vi "Queue_Enqueue.vi"(6 "data":variant, 7 "timeout (-1)":i32=-1, 9 "cmd":string, 10 "queue":refnum<queue>) -> (1 "error out":errorcluster, 2 "queue out":refnum<queue>)   [LabVIEW 2009]
uses:
  Queue_Type.ctl
panel:
  in  "error in (no error)":errorcluster
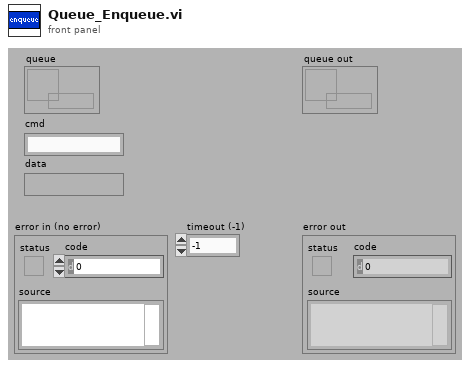
[diagram p1: front panel]
types:
  T1 = typedef "Queue_Type.ctl" = cluster{"cmd":string, "data":variant}
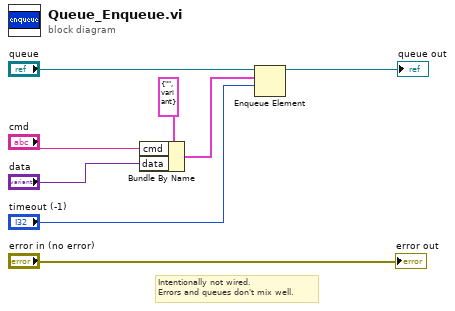
[diagram p0: block diagram]
diagram:
  # "Intentionally not wired.\nErrors and queues don't mix well."
  n1 = Bundle By Name(cluster=T1 {"cmd"="", "data"=variant} ("Queue type"), "cmd"="cmd", "data"="data") -> (w4:T1)
  n2 = Enqueue Element(queue="queue", element=w4, timeout in ms (-1)="timeout (-1)") -> (queue out=→"queue out":refnum<queue>)  [unwired: 1 in, 2 out]
  "error out" <- "error in (no error)"
